vi "GetRectangleBound.vi"(8 "error in (no error)":errorcluster, 10 "Point":refnum<class "Point.lvclass">, 11 "Rectangle in":refnum<class "Rectangle.lvclass">) -> (0 "error out":errorcluster, 2 "rect":T1, 3 "Rectangle out":refnum<class "Rectangle.lvclass">)   [LabVIEW 2021, in "Picture2D.lvlib" / "Rectangle.lvclass"]
uses:
  Rectangle.lvclass
  Point/Point.lvclass
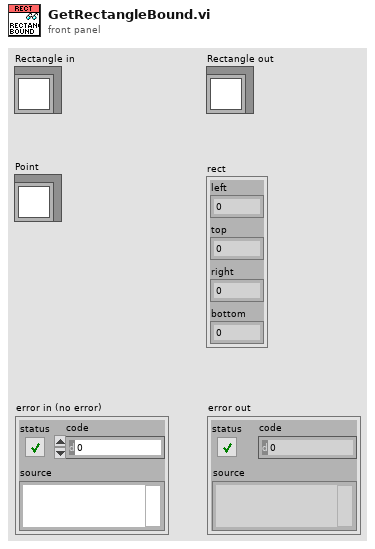
[diagram p1: front panel]
types:
  T1 = cluster{"left":i16, "top":i16, "right":i16, "bottom":i16}
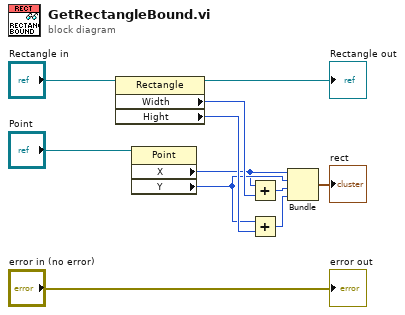
[diagram p0: block diagram]
diagram:
  n1 = property class="Rectangle"(reference="Rectangle in") -> (reference out=→"Rectangle out":refnum<class "Rectangle.lvclass">, "Width"=w10:i16, "Hight"=w11:i16)  [unwired: 1 in, 1 out]
  n2 = property class="Point"(reference="Point") -> ("X"=w4:i16, "Y"=w5:i16)  [unwired: 1 in, 2 out]
  n3 = Add(x=w4, y=w10) -> (x+y=w6:i16)
  n4 = Add(x=w5, y=w11) -> (x+y=w7:i16)
  n5 = Bundle("X"=w4, "Y"=w5, w6, w7) -> (→"rect":cluster{"X":i16, "Y":i16, i16, i16})  [unwired: 1 in]
  "error out" <- "error in (no error)"
